vi "combine1dArrays.vi"(11 "Array In":dbl[](array[numeric])) -> (3 "Array Out":dbl[](array[numeric]))   [LabVIEW 2013]
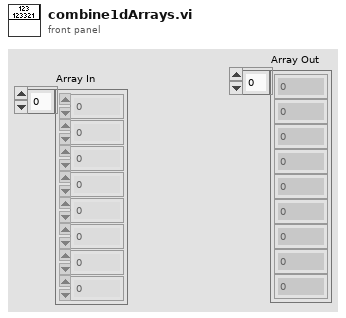
[diagram p1: front panel]
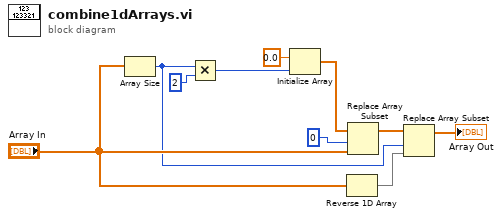
[diagram p0: block diagram]
diagram:
  n1 = Array Size(array="Array In") -> (size(s)=w3:i32)
  n2 = Multiply(x=w3, y=2) -> (x*y=w6:i32)
  n3 = Initialize Array(0.0 ("element"), w6) -> (w8:dbl[])
  n4 = Reverse 1D Array(array="Array In") -> (reversed array=w4:dbl[])
  n5 = Replace Array Subset(array=w8, new element="Array In", index=0) -> (w2:dbl[])
  n6 = Replace Array Subset(array=w2, new element=w4, index=w3) -> (→"Array Out":dbl[])
